vi "action.vi"(0 "HGF_Visitor in":refnum<class "HGF_Visitor.lvclass">, 2 "HGF_Visitable":refnum<class "HGF_Visitable.lvclass">, 5 "error in (no error)":errorcluster) -> (14 "HGF_Visitor out":refnum<class "HGF_Visitor.lvclass">, 16 "dup HGF_Visitable":refnum<class "HGF_Visitable.lvclass">, 19 "error out":errorcluster)   [LabVIEW 2014, in "HGF_BaseClasses.lvlib" / "HGF_Visitor.lvclass"]
doc: "This is a dynamic dispatch VI that is called from Visitor.visit(). It will call member VIs of Visitable to perform the requested action which means: calling public methods of Visitable child class.\n\n<B>Hint:</B> This method is abstract and need to be implemented by child classes."
uses:
  HGF_Visitor.lvclass
  HGF_Auxiliary/HGF_Auxiliary.lvlib
  HGF_Auxiliary/ErrorCode.ctl
  HGF_Auxiliary/Severity.ctl
  HGF_Visitable/HGF_Visitable.lvclass
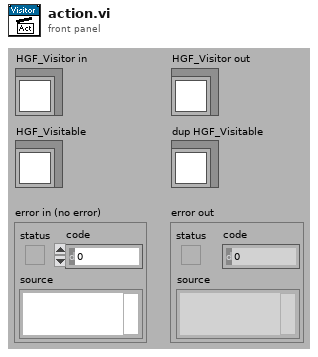
[diagram p1: front panel]
types:
  T1 = typedef "HGF_Auxiliary.lvlib/Severity.ctl" = enum16{"Info", "Warning", "Fault", "Error", "Fatal"}
  T2 = typedef "HGF_Auxiliary.lvlib/ErrorCode.ctl" = enum32{"No error", "Function not supported.", "This VI is for friends only.", "Reference object aready exisits.", "Parameter out of range.", "Not a rendezvous.", "Invalid notifier reference.", "Invalid queue reference.", "Self-Test not supported.", "Reset not supported.", "IDN query not supported.", "Error query not supported.", "Incorrect addressee.", "Object already exists.", "No class name specified", "Driver not supported", "Attribute is not writable"}
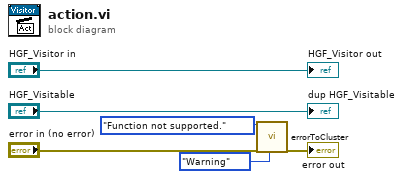
[diagram p0: block diagram]
diagram:
  n1 = call "errorToCluster.vi"("error code"=ErrorCode."Function not supported.", "error in (no error)"="error in (no error)", "severity (Error)"=Severity."Warning") -> ("error out"=→"error out":errorcluster)  [unwired: 2 in, 14 out]
  "HGF_Visitor out" <- "HGF_Visitor in"
  "dup HGF_Visitable" <- "HGF_Visitable"
